vi "XML Parse DBL Range.vi"(3 "Attribut Name":string, 7 "XML Response":string, 8 "Anzahl Elemente":i32) -> (0 "Werte":dbl[](array[numeric]), 2 "XML Response gekürzt":string)   [LabVIEW 2020, in "FT-IR.lvlib" / "TOOLweb Interface.lvlib" / "TOOLweb Interface Hilfs-VIs.lvlib"]
doc: "Sucht in dem XML-Poll-Response-String \"XML-Response\" den Eintrag mit dem Elementnamen \"Attribut Name\" und liefert dessen Werte im DBL-Array \"Werte\". \n\nDer Eintrag wird dann entfernt, damit eine weiteres Parser-VI am Ausgang \"XML Response gekürzt\" nicht wieder den ganzen String durchsuchen muss."
uses:
  TOOLweb Interface Hilfs-VIs.lvlib
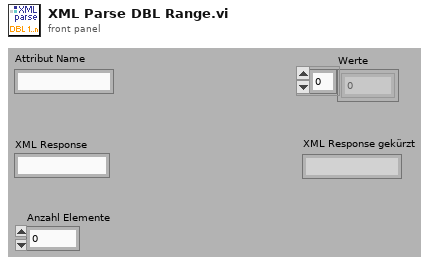
[diagram p1: front panel]
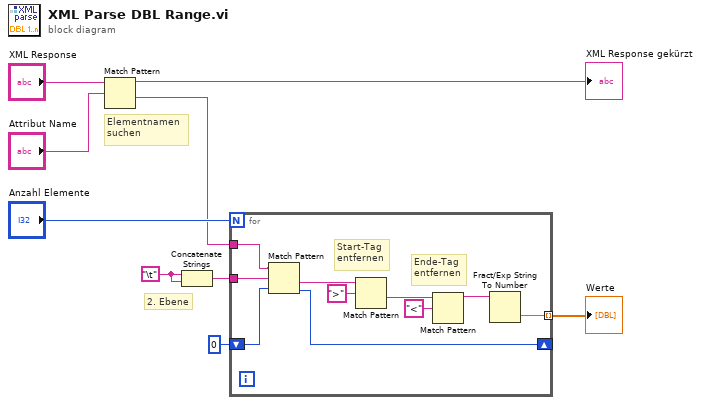
[diagram p0: block diagram]
diagram:
  w6 = "\t"
  # "2. Ebene"
  # "Elementnamen\nsuchen"
  n1 = Match Pattern(string="XML Response", regular expression="Attribut Name") -> (before substring=→"XML Response gekürzt":string, after substring=w1:string)  [unwired: 3 out]
  n2 = Concatenate Strings(w6, w6) -> (w5:string)
  n3 = for {
    N: "Anzahl Elemente" -> [_]
    tunnel: w1 -> [w19]
    tunnel: w5 -> [w18]
    shift-right: [w16] -> _
    shift-left: 0 ("offset past match") -> [w17]
    tunnel: [w11] -> w2 mode=indexing
    # "Start-Tag\nentfernen"
    # "Ende-Tag\nentfernen"
    n4 = Match Pattern(string=w19, regular expression=w18, offset (0)=w17) -> (after substring=w15:string, offset past match=w16:i32)  [unwired: 2 out]
    n5 = Match Pattern(string=w15, regular expression=">" ("Regulärer Ausdruck")) -> (after substring=w12:string)  [unwired: 4 out]
    n6 = Match Pattern(string=w12, regular expression="<" ("Regulärer Ausdruck")) -> (before substring=w10:string)  [unwired: 4 out]
    n7 = Fract/Exp String To Number(string=w10) -> (number=w11:dbl)  [unwired: 4 out]
  }
  "Werte" <- w2
